vi "Generate Toggle DO DAQ Out Cmd Event.vi"(4 "mode (manual)":T1, 6 "WaitTime (20ms)":u32=20, 7 "ToggleInterval (250ms)":u32=250, 8 "error in (no error)":errorcluster, 9 "BoolState":bool, 10 "DO IOName":string, 11 "DAQ":refnum<class "DAQ.lvclass">) -> (0 "error out":errorcluster, 3 "DAQ":refnum<class "DAQ.lvclass">)   [LabVIEW 2017, in "DAQ.lvclass"]
doc: "Developed by Kevin Thompson\nkevin@thompsonengineering.net\n\nCopyright 2018-2020\nThompson Engineering, LLC"
uses:
  DAQ.lvclass
  DataTypes/TD DAQ Output EventSenderMode-enum.ctl
  Process/ProcessSupport/TD DAQ Output Cmd EventData--cluster.ctl
  Process/ProcessSupport/TD DaqOutCmd--enum.ctl
  DAQ.lvclass/DAQ.ctl
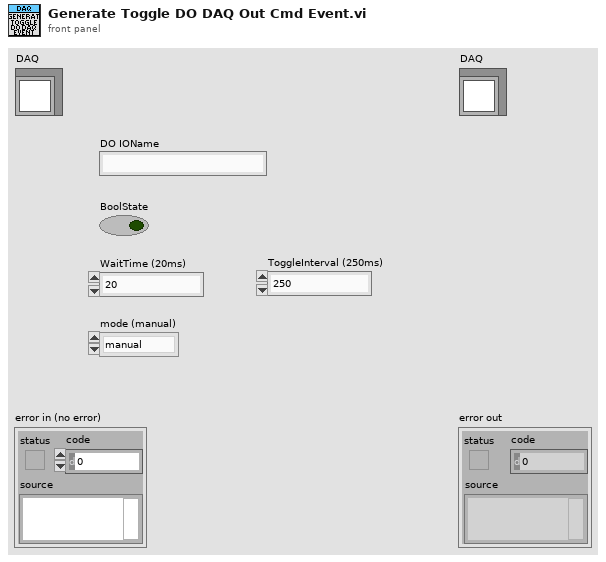
[diagram p1: front panel]
types:
  T1 = typedef "DAQ.lvclass/TD DAQ Output EventSenderMode-enum.ctl" = enum16{"manual", "automation"}
  T2 = typedef "DAQ.lvclass/TD DaqOutCmd--enum.ctl" = enum16{"Set DO", "Set AO", "Toggle DO"}
  T3 = typedef "DAQ.lvclass/TD DAQ Output Cmd EventData--cluster.ctl" = cluster{"TimeStamp":dbl, "DaqOutCmd":T2, "IOName":string, "BoolState":bool, "AnalogVal":dbl, "WaitTime (ms)":u32, "mode":T1, "vData":variant}
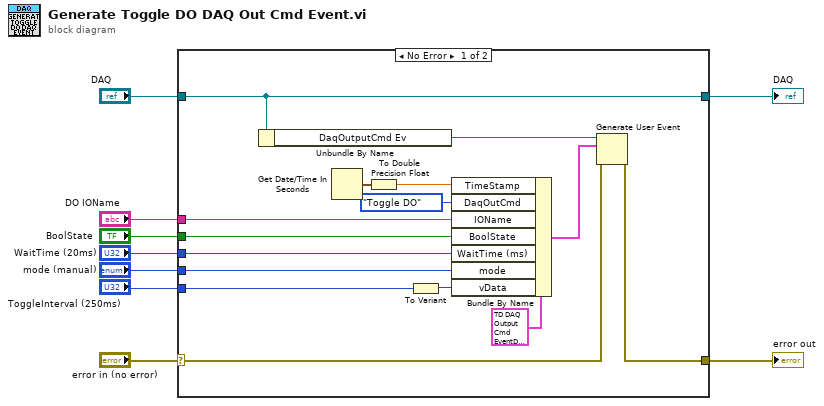
[diagram p0: block diagram]
diagram:
  n1 = case shown="No Error" "error in (no error)" {
    selector: "error in (no error)" -> [w16 w26]
    tunnel: [w15 w26] -> w8
    tunnel: [w24 w25] -> w6
    tunnel: "DAQ" -> [w24 w25]
    tunnel: "DO IOName" -> [w12 _]
    tunnel: "WaitTime (20ms)" -> [w17 _]
    tunnel: "BoolState" -> [w14 _]
    tunnel: "mode (manual)" -> [w13 _]
    tunnel: "ToggleInterval (250ms)" -> [w10 _]
    frame No Error {
      n2 = Unbundle By Name(w24) -> ("DaqOutputCmd Ev"=w23:refnum<user-event>)
      n3 = Get Date/Time In Seconds() -> (seconds since 1Jan1904=w20:timestamp)
      n4 = To Double Precision Float(number=w20) -> (double precision float=w19:dbl)
      n5 = To Variant(anything=w10) -> (Variant=w11:variant)
      n6 = Bundle By Name(cluster=T3 {"TimeStamp"=0.0, "DaqOutCmd"=enum."Set DO", "IOName"="", "BoolState"=FALSE, "AnalogVal"=0.0, "WaitTime (ms)"=0, "mode"=enum."manual", "vData"=variant} ("DaqOutputCmd"), "TimeStamp"=w19, "DaqOutCmd"=TD_DaqOutCmd--enum."Toggle DO", "IOName"=w12, "BoolState"=w14, "WaitTime (ms)"=w17, "mode"=w13, "vData"=w11) -> (w21:T3)
      n7 = Generate User Event(user event=w23, event data cluster=w21, error in=w16) -> (error out=w15:errorcluster)  [unwired: 1 in, 1 out]
    }
    frame Error {
    }
  }
  "error out" <- w8
  "DAQ" <- w6
